vi "Save.vi"(8 "Rising Index 1":i32[](array[numeric]), 9 "Rising Index 2":i32[](array[numeric]), 10 "PMT (AI 0)":u8[](graph), 11 "Save?":bool) -> ()   [LabVIEW 2012]
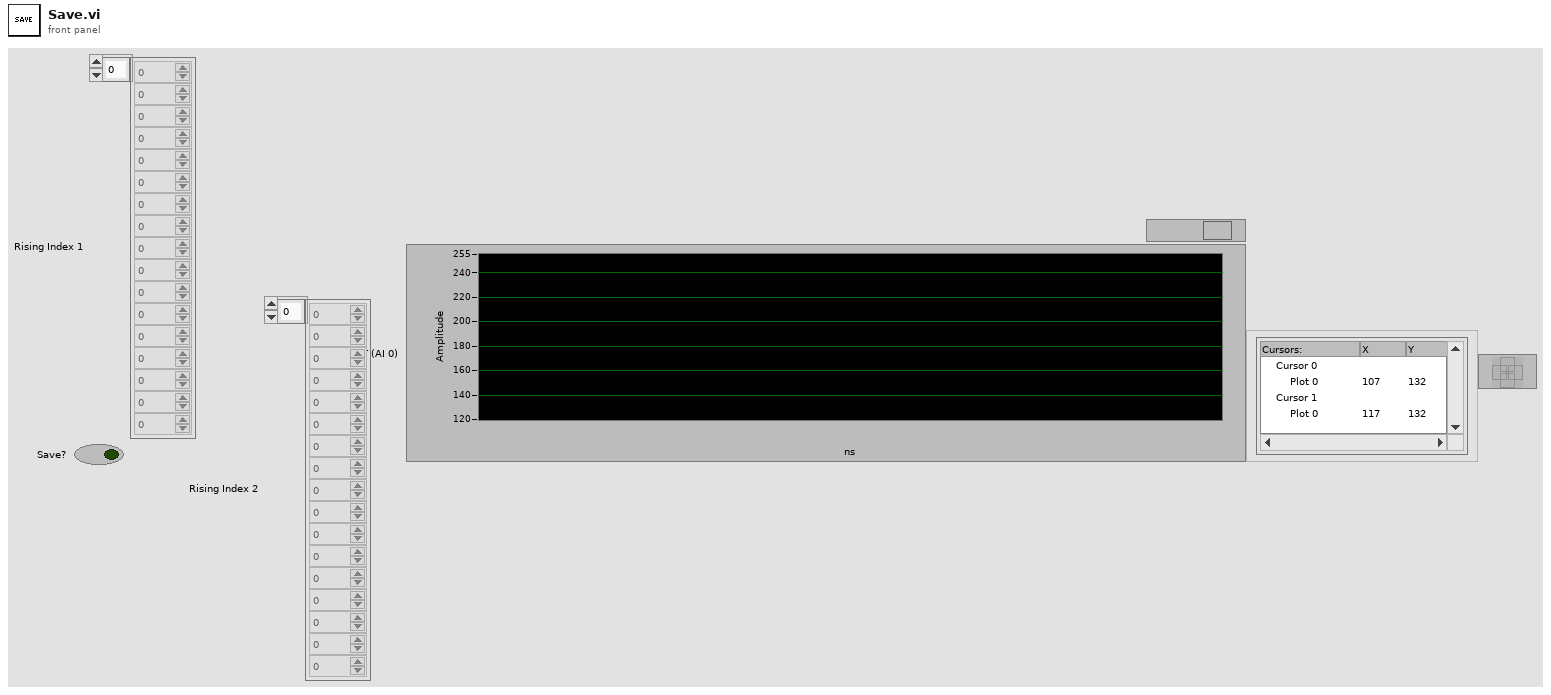
[diagram p1: front panel]
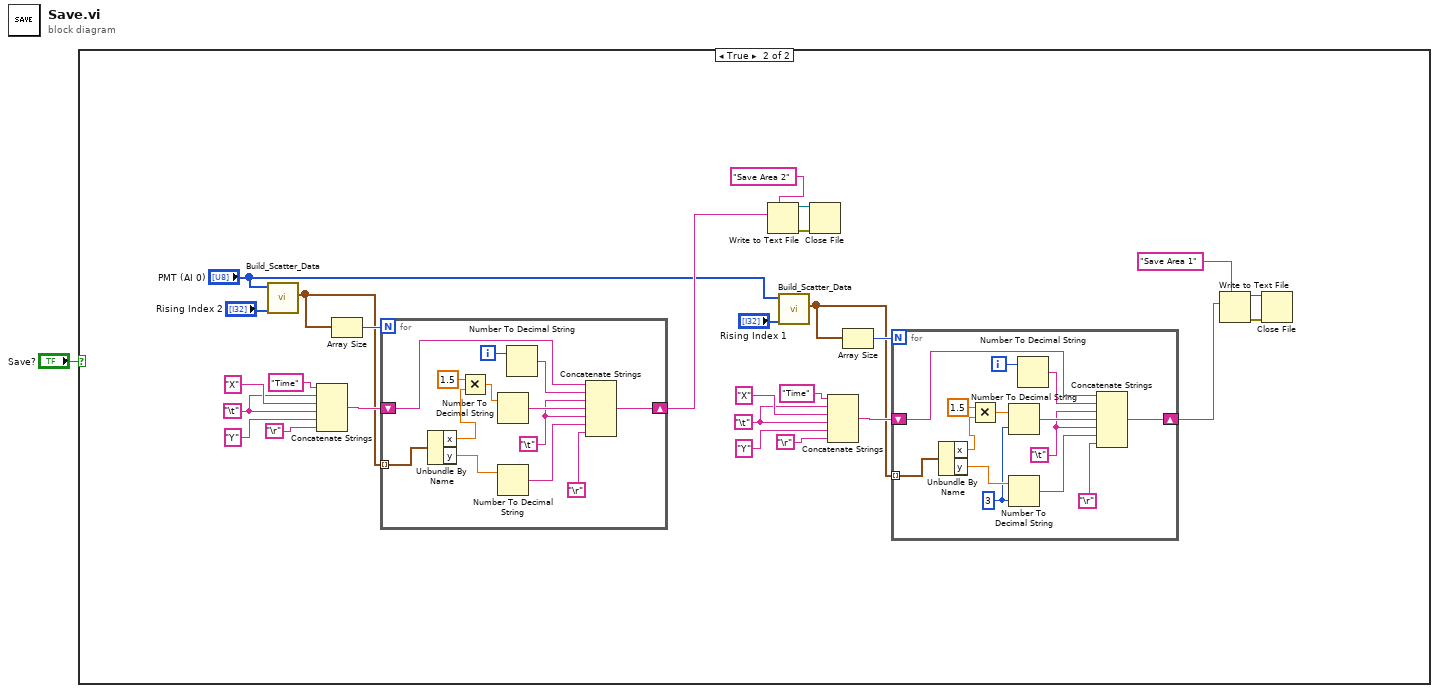
[diagram p0: block diagram]
diagram:
  n1 = case shown="True" "Save?" {
    frame False {
    }
    frame True {
      w10 = "\t"
      w21 = "\t"
      n2 = call "Build_Scatter_Data.vi"("Rising Index"="Rising Index 2", "PMT (AI 0)"="PMT (AI 0)") -> ("data"=w19:cluster{"x":dbl, "y":dbl}[])  [unwired: 9 in]
      n3 = Concatenate Strings("Time", w21, "X", w21, "Y", "\r") -> (w22:string)
      n4 = Array Size(array=w19) -> (size(s)=w24:i32)
      n5 = for {
        N: w24 -> [_]
        shift-right: [w54] -> w23
        shift-left: w22 -> [w55]
        tunnel: w19 -> [w50] mode=indexing
        i -> [w51]
        w47 = "\t"
        n6 = Unbundle By Name(w50) -> ("x"=w44:dbl, "y"=w49:dbl)
        n7 = Multiply(x=1.5, y=w44) -> (x*y=w43:dbl)
        n8 = Number To Decimal String(number=w43) -> (decimal integer string=w48:string)  [unwired: 1 in]
        n9 = Number To Decimal String(number=w49) -> (decimal integer string=w52:string)  [unwired: 1 in]
        n10 = Number To Decimal String(number=w51) -> (decimal integer string=w53:string)  [unwired: 1 in]
        n11 = Concatenate Strings(w55, w53, w47, w48, w47, w52, "\r") -> (w54:string)
      }
      n12 = Write to Text File(prompt (Choose or enter file path)="Save Area 2" ("prompt"), text=w23) -> (refnum out=w28:refnum<file>, error out=w20:errorcluster)  [unwired: 2 in, 1 out]
      n13 = call "Build_Scatter_Data.vi"("Rising Index"="Rising Index 1", "PMT (AI 0)"="PMT (AI 0)") -> ("data"=w9:cluster{"x":dbl, "y":dbl}[])  [unwired: 9 in]
      n14 = Close File(refnum=w28, error in=w20) -> ()  [unwired: 2 out]
      n15 = Concatenate Strings("Time", w10, "X", w10, "Y", "\r") -> (w11:string)
      n16 = Array Size(array=w9) -> (size(s)=w12:i32)
      n17 = for {
        N: w12 -> [_]
        shift-right: [w41] -> w7
        shift-left: w11 -> [w42]
        tunnel: w9 -> [w37] mode=indexing
        i -> [w38]
        w32 = 3
        w34 = "\t"
        n18 = Unbundle By Name(w37) -> ("x"=w30:dbl, "y"=w36:dbl)
        n19 = Multiply(x=1.5, y=w30) -> (x*y=w29:dbl)
        n20 = Number To Decimal String(number=w29, width (-)=w32) -> (decimal integer string=w35:string)
        n21 = Number To Decimal String(number=w36, width (-)=w32) -> (decimal integer string=w39:string)
        n22 = Number To Decimal String(number=w38) -> (decimal integer string=w40:string)  [unwired: 1 in]
        n23 = Concatenate Strings(w42, w40, w34, w35, w34, w39, "\r") -> (w41:string)
      }
      n24 = Write to Text File(prompt (Choose or enter file path)="Save Area 1" ("prompt"), text=w7) -> (refnum out=w18:refnum<file>, error out=w17:errorcluster)  [unwired: 2 in, 1 out]
      n25 = Close File(refnum=w18, error in=w17) -> ()  [unwired: 2 out]
    }
  }
